vi "StopProcesses.vi"(8 "error in (no error)":errorcluster, 9 "timeout in ms (-1)":i32=-1, 11 "JKI SMO in":refnum<class "JKI SMO.lvclass">) -> (0 "error out":errorcluster, 3 "JKI SMO out":refnum<class "JKI SMO.lvclass">)   [LabVIEW 2013, in "JKI SMO.lvclass"]
doc: "Stops all processes in the JKI SMO.\n\n---------------------------------------------------------------\nJKI State Machine Objects™\nhttp://jki.net/state-machine-objects/\nCopyright (C) 2005-2015, JKI <info@jki.net>\nALL RIGHTS RESERVED"
uses:
  JKI SMO.lvclass
  JKI SMO.lvclass/JKI SMO.ctl
  Typedefs/StopProcessEventData--Cluster.ctl
panel:
  # "For instructions on how to use the JKI State Machine Objects, examples and video tutorials, visit:\nhttp://jki.net/state-machine-objects/\n\nJKI State Machine Objects™\nhttp://jki.net/state-machine-objects/\nCopyright (C) 2005-2015, JKI <info@jki.net>\nALL RIGHTS RESERVED"
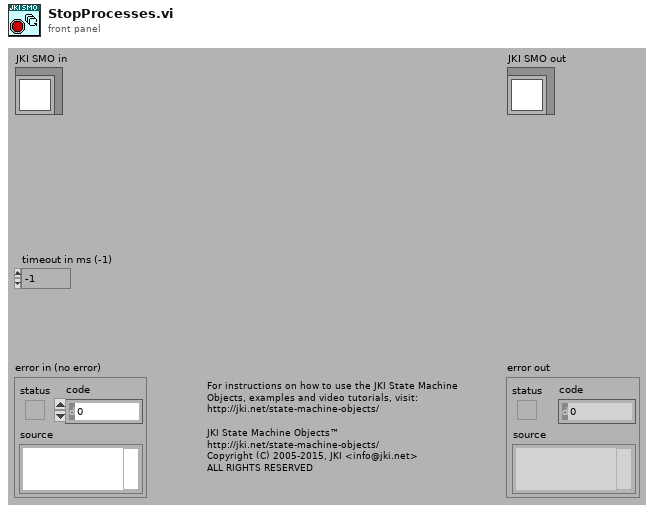
[diagram p1: front panel]
types:
  T1 = typedef "JKI SMO.lvclass/StopProcessEventData--Cluster.ctl" = cluster{"Time Stamp":timestamp}
  T2 = typedef "JKI SMO.lvclass/PrivateData--Cluster.ctl" = cluster{"Processes Clone VI Ref [ ]":refnum<vi>[], "Processes Clone Name [ ]":string[], "Process Sync RendezVous":T3, "Protected Events":T4, "Registered Process [ ]":T5[]}
  T3 = typedef "Rendezvous RefNum" = refnum<k1>
  T4 = typedef "JKI SMO.lvclass/ProtectedEvents--Cluster.ctl" = cluster{"StopProcesses":refnum<user-event>, "AbortProcesses":refnum<user-event>}
  T5 = typedef "JKI SMO.lvclass/RegisteredProcessData--Cluster.ctl" = cluster{"Name":string, "Static VI Ref":refnum<vi>}
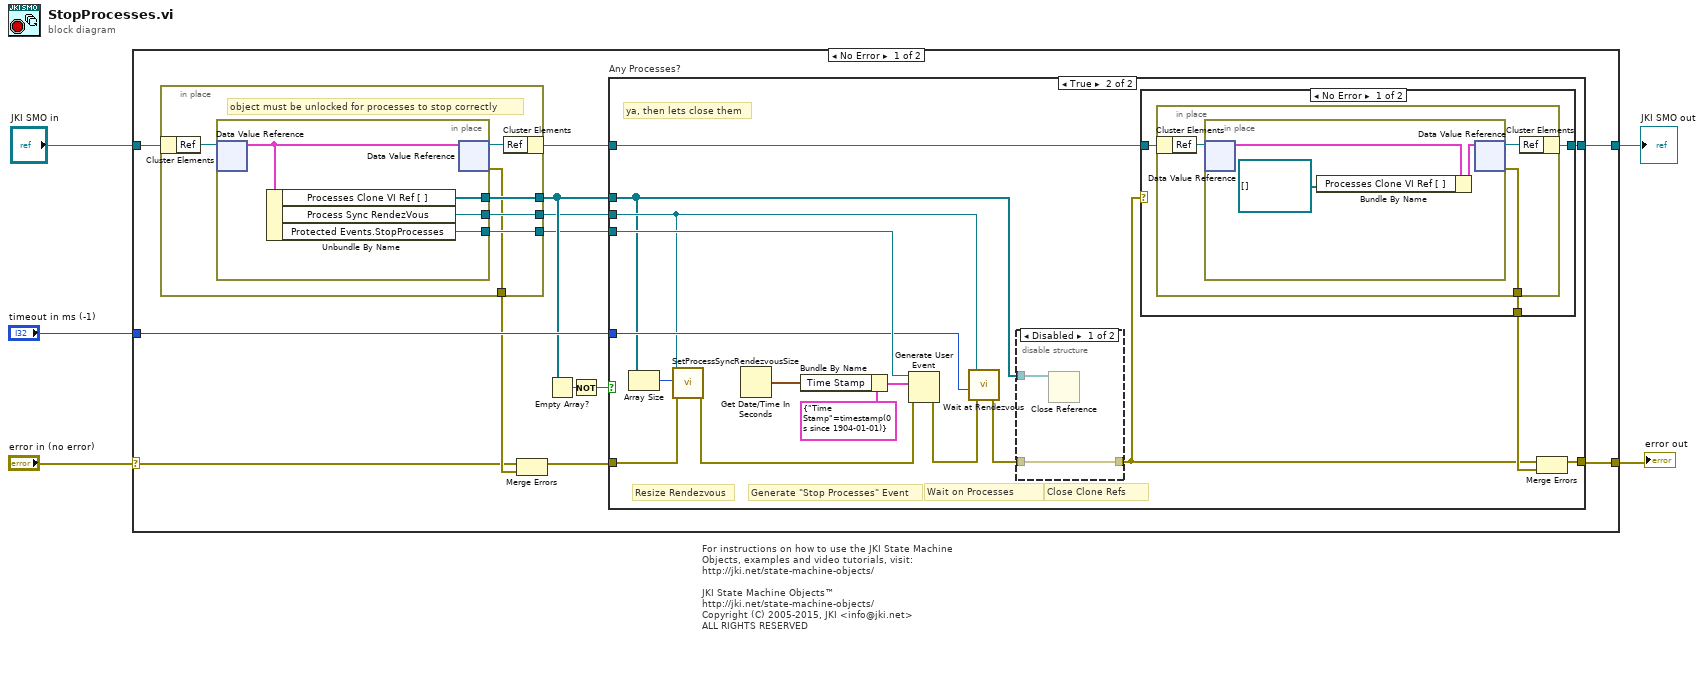
[diagram p0: block diagram]
diagram:
  # "For instructions on how to use the JKI State Machine Objects, examples and video tutorials, visit:\nhttp://jki.net/state-machine-objects/\n\nJKI State Machine Objects™\nhttp://jki.net/state-machine-objects/\nCopyright (C) 2005-2015, JKI <info@jki.net>\nALL RIGHTS RESERVED"
  n1 = case shown="No Error" "error in (no error)" {
    selector: "error in (no error)" -> [w9 w63]
    tunnel: [w17 w63] -> w4
    tunnel: [w6 w62] -> w2
    tunnel: "JKI SMO in" -> [w11 w62]
    tunnel: "timeout in ms (-1)" -> [w18 _]
    frame No Error {
      n2 = in-place {
        in-place-border: [w24] -> w14
        in-place-border: [w23] -> w13
        in-place-border: [w22] -> w12
        in-place-border: [w19] -> w10
        # "object must be unlocked for processes to stop correctly"
        n3 = in-place-cluster #1(w11) -> ("Ref"=w21:refnum<data-value>)
        n4 = in-place {
          in-place-border: [w28] -> w24
          in-place-border: [w27] -> w23
          in-place-border: [w26] -> w22
          n5 = in-place-dvr #2(w21) -> (w25:T2)  [unwired: 1 out]
          n6 = Unbundle By Name(w25) -> ("Processes Clone VI Ref [ ]"=w28:refnum<vi>[], "Process Sync RendezVous"=w27:T3, "Protected Events.StopProcesses"=w26:refnum<user-event>)
          n7 = in-place-dvr #2(w25) -> (w20:refnum<data-value>, w19:errorcluster)
        }
        n8 = in-place-cluster #1("Ref"=w20) -> (w7:refnum<class "JKI SMO.lvclass">)
      }
      n9 = Merge Errors(w9, w10) -> (w8:errorcluster)
      n10 = Empty Array?(array=w14) -> (empty?=w16:bool)
      n11 = Not(x=w16) -> (.not. x?=w15:bool)
      n12 = case "Any Processes?" shown="True" w15 {
        tunnel: w12 -> [_ w47]
        tunnel: w18 -> [_ w46]
        tunnel: [w30 w31] -> w17
        tunnel: w8 -> [w30 w40]
        tunnel: w13 -> [_ w39]
        tunnel: w14 -> [_ w38]
        tunnel: w7 -> [w29 w35]
        tunnel: [w29 w34] -> w6
        frame False {
        }
        frame True {
          # "ya, then lets close them"
          # "Resize Rendezvous"
          # "Close Clone Refs"
          # "Wait on Processes"
          # "Generate \"Stop Processes\" Event"
          n13 = Array Size(array=w38) -> (size(s)=w41:i32)
          n14 = call "SetProcessSyncRendezvousSize.vi"("error in"=w40, "# processes"=w41, "Process Sync Rendezvous"=w39) -> ("error out"=w37:errorcluster)  [unwired: 8 in]
          n15 = Get Date/Time In Seconds() -> (seconds since 1Jan1904=w36:timestamp)
          n16 = Bundle By Name(cluster=T1 {"Time Stamp"=timestamp(0 s since 1904-01-01)} ("event data"), "Time Stamp"=w36) -> (w43:T1)
          n17 = Generate User Event(user event=w47, event data cluster=w43, error in=w37) -> (error out=w42:errorcluster)  [unwired: 1 in, 1 out]
          n18 = call <vilib>:"Wait at Rendezvous.vi"("error in (no error)"=w42, "ms timeout (-1)"=w46, "rendezvous"=w39) -> ("error out"=w45:errorcluster)  [unwired: 4 out]
          n19 = disable-structure shown="Disabled" {
            disable-tunnel: w45 -> [w60 w61]
            disable-tunnel: [w60 w61] -> w32
            disable-tunnel: w38 -> [w59 _]
            frame Disabled {
              n20 = Close Reference(reference=w59) -> ()  [unwired: 1 in, 1 out]
            }
            frame Enabled {
            }
          }
          n21 = case shown="No Error" w32 {
            selector: w32 -> [_ w57]
            tunnel: w35 -> [w50 w58]
            tunnel: [w49 w58] -> w34
            tunnel: [w48 w57] -> w33
            frame No Error {
              n22 = in-place {
                in-place-border: [w51] -> w48
                n23 = in-place-cluster #3(w50) -> ("Ref"=w53:refnum<data-value>)
                n24 = in-place {
                  n25 = in-place-dvr #4(w53) -> (w55:T2)  [unwired: 1 out]
                  n26 = Bundle By Name(cluster=w55, "Processes Clone VI Ref [ ]"=refnum<vi>[] [] ("Process VI References")) -> (w54:T2)
                  n27 = in-place-dvr #4(w54) -> (w52:refnum<data-value>, w51:errorcluster)
                }
                n28 = in-place-cluster #3("Ref"=w52) -> (w49:refnum<class "JKI SMO.lvclass">)
              }
            }
            frame Error {
            }
          }
          n29 = Merge Errors(w32, w33) -> (w31:errorcluster)
        }
      }
    }
    frame Error {
    }
  }
  "error out" <- w4
  "JKI SMO out" <- w2
